vi "Read_Instr.vi"(8 "error in (no error)":errorcluster caption="entrée d'erreur (pas d'erreur)", 11 "Class Uart en entrée":refnum<class "Class Instrument UART.lvclass">) -> (0 "error out":errorcluster caption="sortie d'erreur", 3 "Class Uart en Sortie":refnum<class "Class Instrument UART.lvclass">)   [LabVIEW 2020, in "Library Instrument & Equipement.lvlib" / "Library Instruments.lvlib" / "Class Instrument UART.lvclass"]
uses:
  Class Instrument UART.lvclass
  Class Instrument UART.lvclass/Class Instrument UART.ctl
  Instrument (Default)/Class Instrument (Default).lvclass
  UART/UART (Default)/Class UART (Default).lvclass
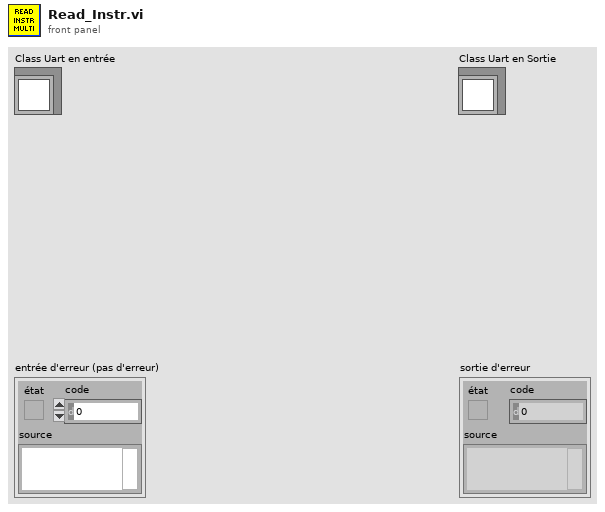
[diagram p1: front panel]
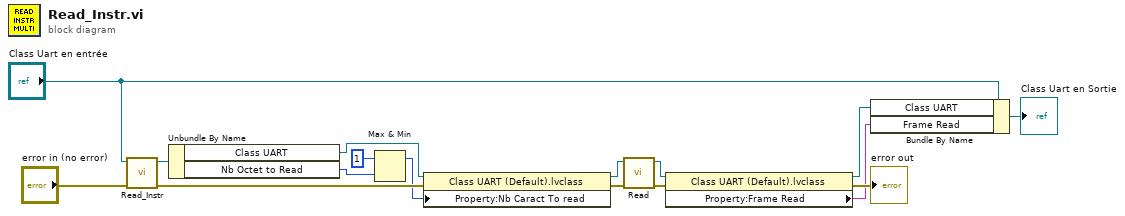
[diagram p0: block diagram]
diagram:
  n1 = call-parent "Read_Instr.vi"("error in (no error)"="error in (no error)", "Class Instrument (Default) en entrée"="Class Uart en entrée") -> ("error out"=w5:errorcluster, "Class Instrument (Default) en sortie"=w15:refnum<class "Class Instrument UART.lvclass">)  [unwired: 8 in]
  n2 = Unbundle By Name(w15) -> ("Class UART"=w7:refnum<class "Class UART (Default).lvclass">, "Nb Octet to Read"=w2:u16)
  n3 = Max & Min(x=u16 1, y=w2) -> (max(x,y)=w1:u16)  [unwired: 1 out]
  n4 = property class="Class UART (Default).lvclass"(reference=w7, error in=w5, "Property:Nb Caract To read"=w1) -> (reference out=w6:refnum<class "Class UART (Default).lvclass">, error out=w4:errorcluster)
  n5 = call-dynamic "Read.vi"("error in (no error)"=w4, "Class UART (Default) en entrée"=w6) -> ("error out"=w10:errorcluster, "Class UART (Default) en sortie"=w12:refnum<class "Class UART (Default).lvclass">)  [unwired: 8 in]
  n6 = property class="Class UART (Default).lvclass"(reference=w12, error in=w10) -> (reference out=w11:refnum<class "Class UART (Default).lvclass">, error out=→"error out":errorcluster, "Property:Frame Read"=w8:string)
  n7 = Bundle By Name(cluster="Class Uart en entrée", "Class UART"=w11, "Frame Read"=w8) -> (→"Class Uart en Sortie":refnum<class "Class Instrument UART.lvclass">)
